vi "Set Volume.vi"(8 "error in (no error)":errorcluster, 10 "Target Volume (ul)":i32, 11 "PHD Ultra in":refnum<class "cetoni.lvclass">) -> (0 "error out":errorcluster, 3 "PHD Ultra out":refnum<class "cetoni.lvclass">)   [LabVIEW 2018, in "cetoni.lvlib" / "cetoni.lvclass"]
uses:
  cetoni.lvclass
  cetoni.lvclass/cetoni.ctl
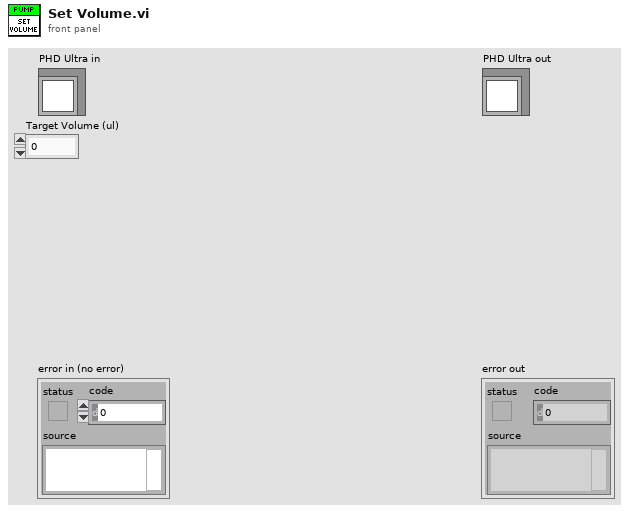
[diagram p1: front panel]
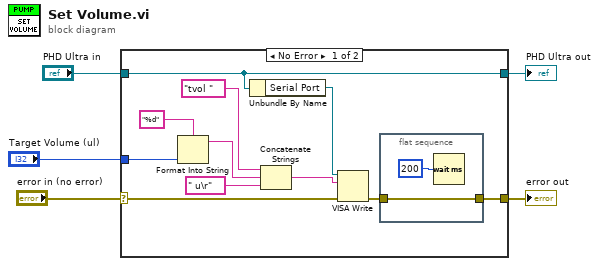
[diagram p0: block diagram]
diagram:
  n1 = case shown="No Error" "error in (no error)" {
    selector: "error in (no error)" -> [w14 w20]
    tunnel: [w6 w20] -> w4
    tunnel: [w16 w19] -> w2
    tunnel: "PHD Ultra in" -> [w16 w19]
    tunnel: "Target Volume (ul)" -> [w9 _]
    frame No Error {
      n2 = Format Into String(format string="%d", w9) -> (resulting string=w11:string)  [unwired: 2 in, 1 out]
      n3 = Unbundle By Name(w16) -> ("Serial Port"=w15:refnum<visa-resource-name>)
      n4 = Concatenate Strings("tvol " ("write buffer"), w11, " u\r" ("write buffer")) -> (w8:string)
      n5 = VISA Write(VISA resource name=w15, write buffer=w8, error in (no error)=w14) -> (error out=w7:errorcluster)  [unwired: 2 out]
      n6 = flat-sequence {
        tunnel: w7 -> [w18]
        tunnel: [w18] -> w6
        frame #0 {
          n7 = Wait (ms)(milliseconds to wait=u32 200) -> ()  [unwired: 1 out]
        }
      }
    }
    frame Error {
    }
  }
  "error out" <- w4
  "PHD Ultra out" <- w2
